vi "udp_server_test.vi"() -> ()   [LabVIEW 2018]
panel:
  out "Ref Array 2":dbl[](array[numeric])=[0.0, 0.0, 0.0, 0.0, 6000.0]
  out "arr sz":i32
  out "data":string
  in  "listening port":u16=60006
  out "client IP address":string
  out "client port":u16
  out "No error":bool
  out "Ref Array":dbl[](array[numeric])=[0.0, 0.0, 0.0, 0.0, 6000.0]
  in  "Stop Program":bool
  # "UDP server test (receive)"
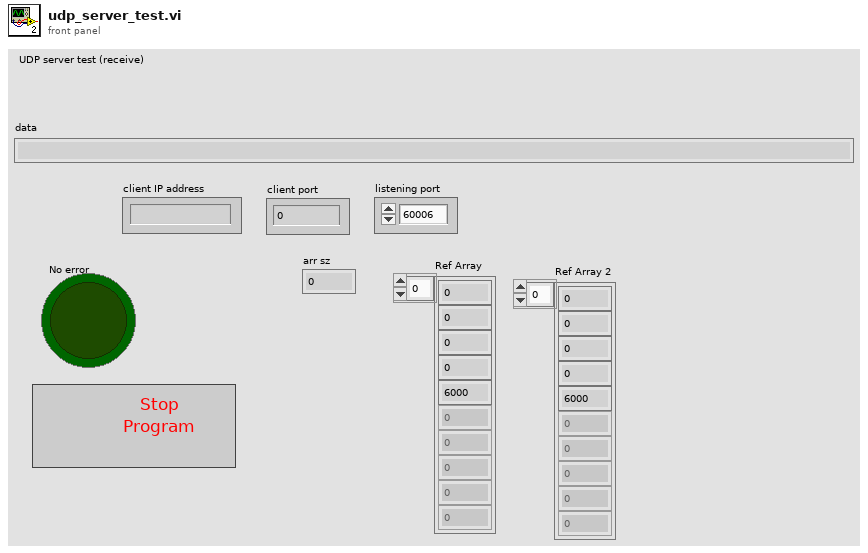
[diagram p1: front panel]
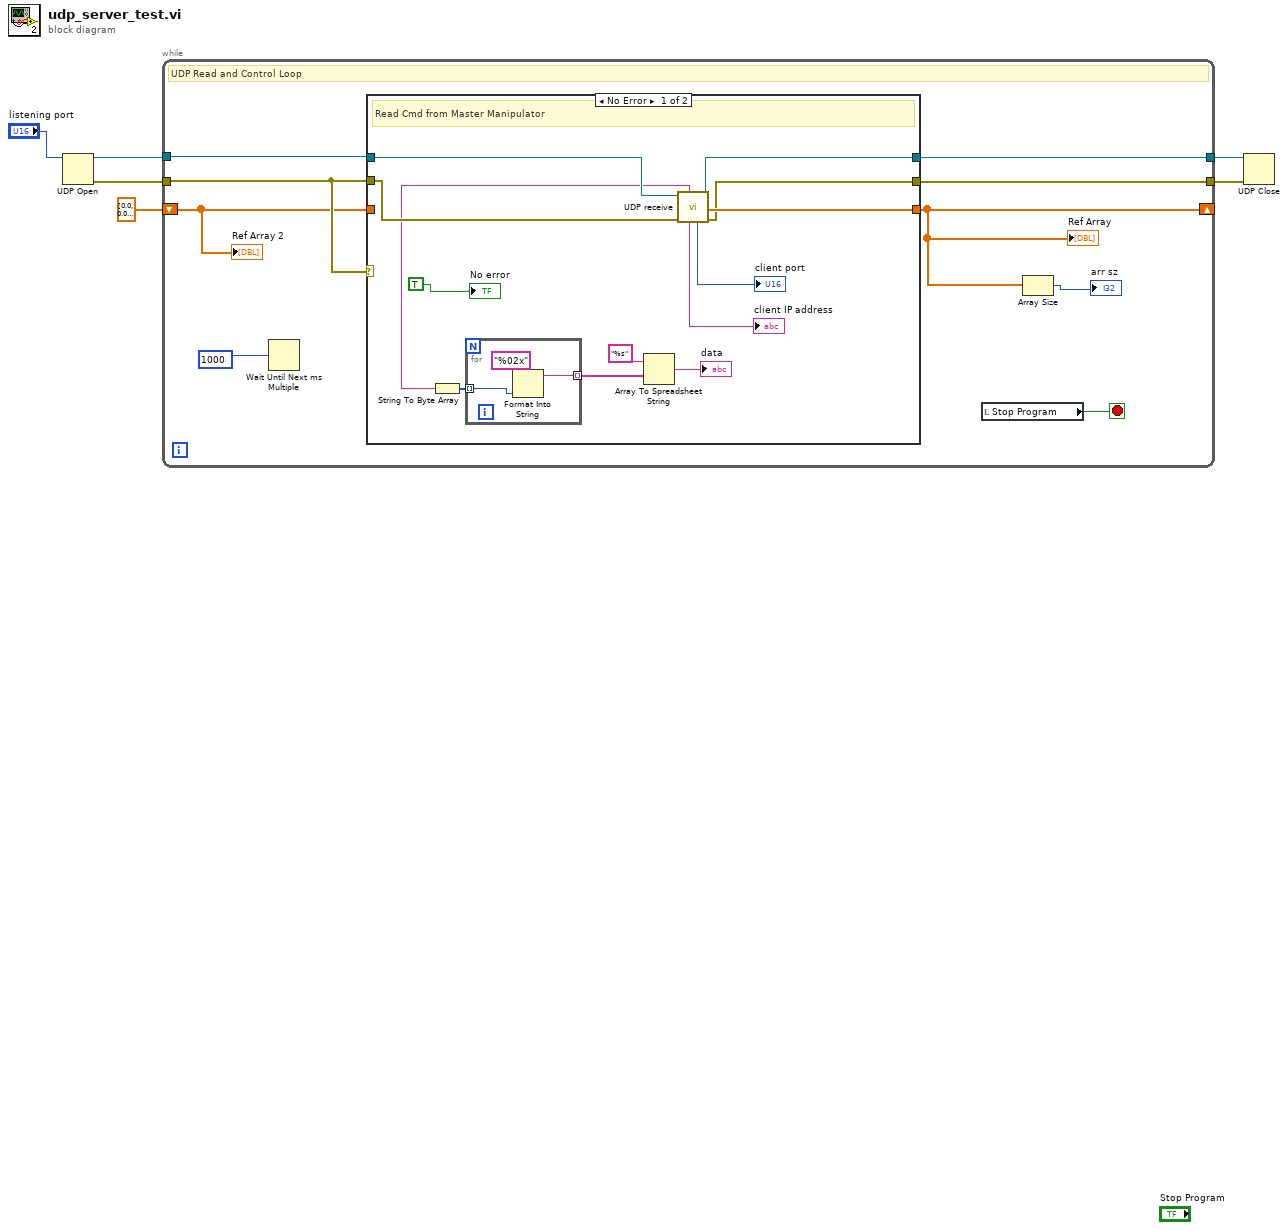
[diagram p0: block diagram]
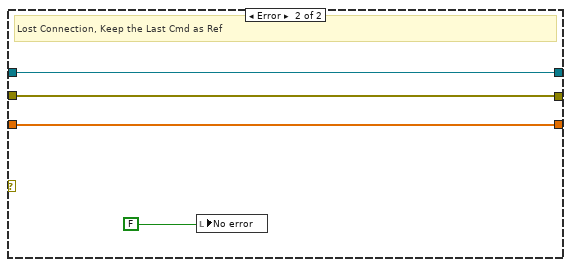
[diagram p2: hidden frame]
diagram:
  n1 = UDP Open(11:"listening port") -> (port=w3:refnum<k16>, 0:w2:errorcluster)  [unwired: 4 in, 1 out]
  n2 = while {
    tunnel: w3 -> [w14]
    tunnel: w2 -> [w11]
    tunnel: [w12] -> w6
    tunnel: [w13] -> w5
    shift-right: [w8] -> _
    shift-left: dbl[] [0.0, 0.0, 0.0, 0.0, 0.0] -> [w7]
    stop <- w15 stop-if-true
    # "UDP Read and Control Loop"
    n3 = Wait Until Next ms Multiple(millisecond multiple=1000) -> ()  [unwired: 1 out]
    n4 = case shown="No Error" w11 {
      tunnel: w14 -> [w20 w35]
      tunnel: w11 -> [w21 w34]
      tunnel: [w23 w33] -> w8
      tunnel: [w19 w35] -> w13
      tunnel: [w22 w34] -> w12
      tunnel: w7 -> [_ w33]
      frame No Error {
        # "Read Cmd from Master Manipulator"
        n5 = call "UDP receive.vi"("error in"=w21, "UDP connection ID"=w20) -> ("error out"=w22:errorcluster, "Array01"=w23:dbl[], "UDP connection ID out"=w19:refnum<k16>, "client port"=→"client port":u16, "client IP address"=→"client IP address":string, "raw data"=w16:string)  [unwired: 4 in]
        n6 = String To Byte Array(string=w16) -> (unsigned byte array=w27:u8[])
        n7 = for {
          tunnel: w27 -> [w31] mode=indexing
          tunnel: [w30] -> w26 mode=indexing
          n8 = Format Into String(format string="%02x", w31) -> (resulting string=w30:string)  [unwired: 2 in, 1 out]
        }
        n9 = Array To Spreadsheet String(array=w26, 3:"%s") -> (spreadsheet string=→"data":string)  [unwired: 1 in]
        "No error" <- TRUE
      }
      frame Error {
        # "Lost Connection, Keep the Last Cmd as Ref"
        n10 = local write "No error"(FALSE) -> ()
      }
    }
    "Ref Array" <- w8
    n11 = local read "Stop Program"() -> (w15:bool)
    n12 = Array Size(array=w8) -> (size(s)=→"arr sz":i32)
    "Ref Array 2" <- w7
  }
  n13 = UDP Close(connection ID=w5, 8:w6) -> ()  [unwired: 2 out]
